vi "fpga_Resampling (P Class_60Hz).vi"(0 "signal in":fxp<+/-,24,1>, 1 "number of channels":T2=7 items=["1"=1, "2"=2, "3"=3, "4"=4, "5"=5, "6"=6, "7"=7, "8"=8, "9"=9, "10"=10, "11"=11, "12"=12, "13"=13, "14"=14, "15"=15, "16"=16], 5 "timestamp [s]":fxp<+,64,32> format="%.42g", 7 "reference channel index":u8, 9 "input valid? (T)":bool=TRUE, 12 "ready for output? (T)":bool=TRUE, 13 "samples per cycle":u16=192) -> (4 "resampled data":T1, 6 "freq time difference":fxp<+,18,-4>, 10 "output valid?":bool, 14 "ready for input?":bool, 15 "error":i32)   [LabVIEW 2013, in "NI_EP_PMU_FPGA.lvlib"]
doc: "Resamples even-time-spaced voltage and current signals into even-angle-spaced signals. The input signals must have a sampling rate of 50 kHz. The output signals are synchronous to the line frequency with a constant number of samples per cycle. Use the Resampling for Power Quality VI if you want to perform resampling on the host computer."
uses:
  <vilib>/addons/Electrical Power/PMU/NI_EP_PMU_FPGA.lvlib
  <vilib>/addons/Electrical Power/PQ/Resampling/FPGA/subVIs/fpga_NofCH.ctl
  <vilib>/addons/Electrical Power/PQ/Resampling/FPGA/subVIs/fpga_Resampled.ctl
  <vilib>/addons/Electrical Power/PQ/Resampling/FPGA/subVIs/fpga_Typedef Fnom.ctl
  <vilib>/addons/Electrical Power/PQ/Resampling/NI_EP_Resample_FPGA.lvlib
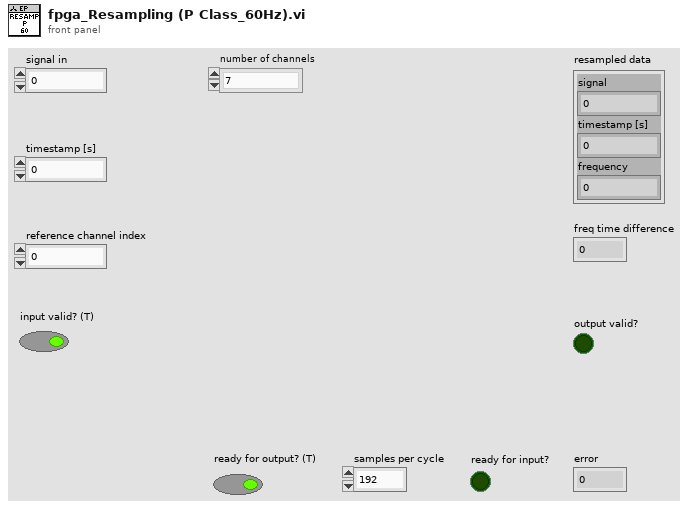
[diagram p1: front panel]
types:
  T1 = typedef "NI_EP_Resample_FPGA.lvlib/fpga_Resampled.ctl" = cluster{"signal":fxp<+/-,32,3>, "timestamp [s]":fxp<+,64,32>, "frequency":fxp<+,32,8>}
  T2 = typedef "NI_EP_Resample_FPGA.lvlib/fpga_NofCH.ctl" = u8
  T3 = typedef "NI_EP_Resample_FPGA.lvlib/fpga_Typedef Fnom.ctl" = u8
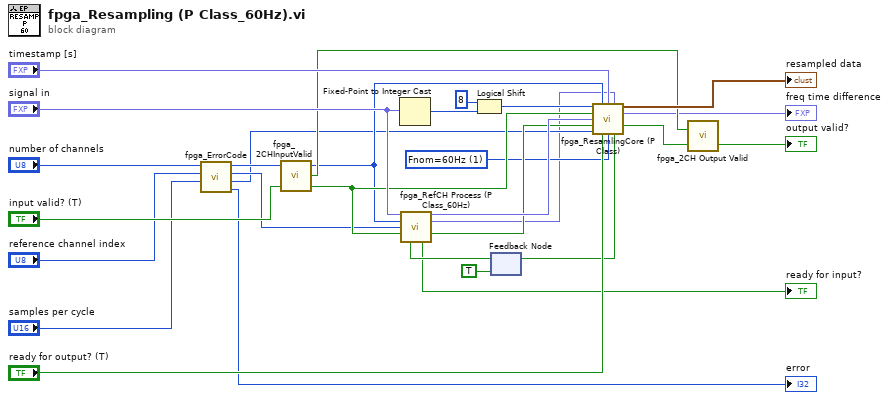
[diagram p0: block diagram]
diagram:
  w6 = T3 1 items=["Fnom=50Hz", "Fnom=60Hz"] ("Fnom")
  n1 = call <vilib>:"fpga_ErrorCode.vi"("samples per cycle"="samples per cycle", "reference channel index"="reference channel index", "number of channels"="number of channels") -> ("error"=→"error":i32, "samples per cycle out"=w7:u16, "ref channel index out"=w8:u8, "number of CH out"=w9:u8)  [unwired: 5 in]
  n2 = call <vilib>:"fpga_2CHInputValid.vi"("input data valid"="input valid? (T)", "Channel number"=w9) -> ("input valid"=w17:bool, "1CH?"=w19:bool, "Channel number"=w10:u8)  [unwired: 1 in]
  n3 = Fixed-Point to Integer Cast(1:"signal in") -> (0:w12:i32)
  n4 = Logical Shift(y=i8 8, x=w12) -> (x << y=w11:i32)
  n5 = feedback #1(TRUE ("Ready for reference input")) -> (w16:bool)
  n6 = call <vilib>:"fpga_RefCH Process (P Class_60Hz).vi"("data in <?24.1>"="signal in", "Channel number"=w10, "Reference index"=w8, "input data valid"=w17, "ready for output"=w16) -> ("Filtered Resampling Ref data"=w15:fxp<+/-,24,3>, "measured frequency"=w3:fxp<+,32,8>, "output valid"=w14:bool, "ready for input"=→"ready for input?":bool)  [unwired: 7 in]
  n7 = call <vilib>:"fpga_ResamlingCore (P Class).vi"("data in"=w11, "Channel number"=w10, "timestamp"="timestamp [s]", "measured frequency"=w3, "input data valid"=w17, "resampling reference in"=w15, "input rs reference valid"=w14, "interpolation factor"=w7, "Ready for output"="ready for output? (T)", "Fnom"=w6) -> ("Resample data and time"=→"resampled data":T1, "freq time difference"=→"freq time difference":fxp<+,18,-4>, "output valid"=w18:bool, "Ready for reference input"=w21:bool)  [unwired: 2 out]
  n8 = feedback-in #1(w21) -> ()
  n9 = call <vilib>:"fpga_2CH Output Valid.vi"("output valid"=w18, "1CH?"=w19) -> ("output valid"=→"output valid?":bool)  [unwired: 1 in]
